vi "relay_block4.vi"(8 "error in":errorcluster, 11 "Modbus master in":refnum<class "Modbus Master.lvclass">) -> (0 "error out":errorcluster, 3 "Modbus master out":refnum<class "Modbus Master.lvclass">)   [LabVIEW 2020]
uses:
  <vilib>/NI/Modbus Library/API/Master/Modbus Master.lvclass
  C:/Program Files/National Instruments/LabVIEW 2020/vi.lib/NI/Modbus Library/API/Modbus API.lvclass
  <vilib>/NI/Modbus Library/API/Modbus API.lvclass/Modbus API.ctl
  <vilib>/NI/Modbus Library/Transmission Data Unit/Transmission Data Unit.lvclass/Transmission Data Unit.ctl
  <vilib>/NI/Modbus Library/Transmission Data Unit/Write Unit ID.vi
  <vilib>/NI/Modbus Library/API/Read Transmission Data Unit.vi
  <vilib>/NI/Modbus Library/API/Write Transmission Data Unit.vi
  status/emergency stop.vi
panel:
  out "current time 2":timestamp
  out "current time":timestamp
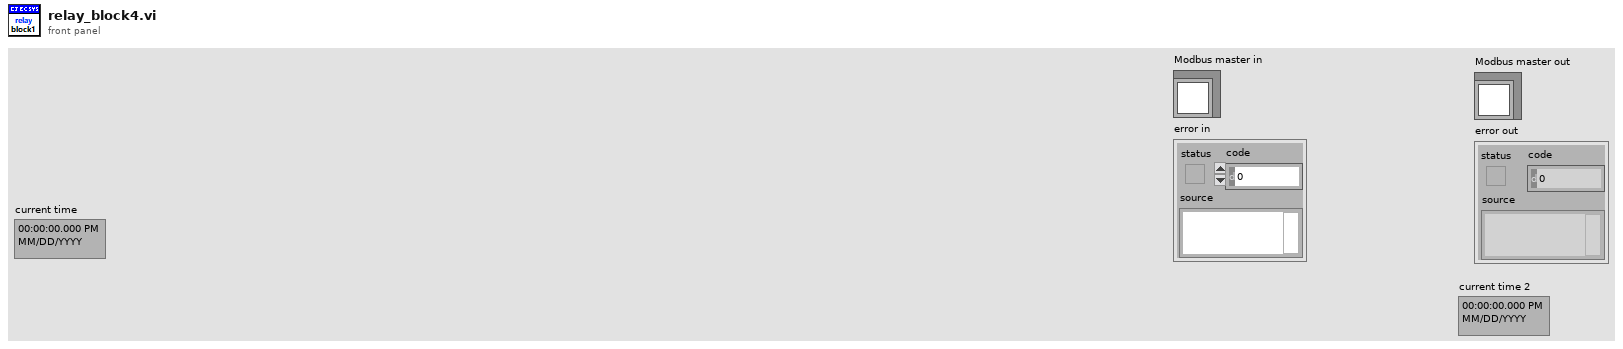
[diagram p1: front panel]
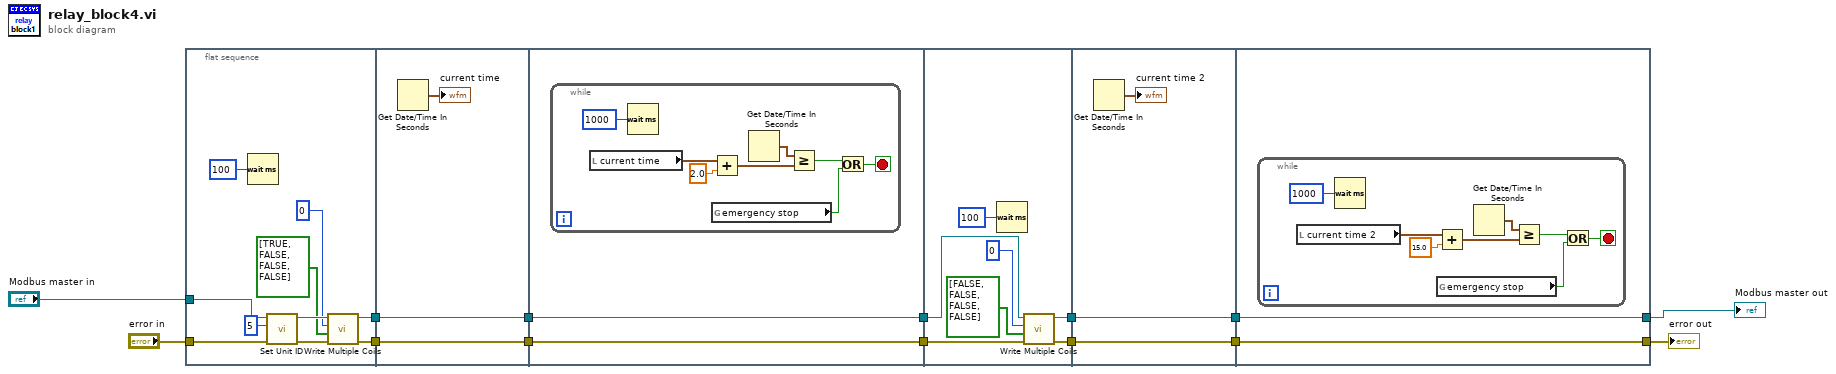
[diagram p0: block diagram]
diagram:
  n1 = flat-sequence {
    tunnel: "Modbus master in" -> [w19]
    tunnel: "error in" -> [w18]
    tunnel: [w17] -> w12
    tunnel: [w16] -> w7
    tunnel: w12 -> [w26]
    tunnel: [w26] -> w11
    tunnel: [w25] -> w8
    tunnel: w7 -> [w25]
    tunnel: w11 -> [w29]
    tunnel: [w29] -> w10
    tunnel: [w28] -> w9
    tunnel: w8 -> [w28]
    tunnel: w10 -> [w41]
    tunnel: w9 -> [w40]
    tunnel: [w39] -> w5
    tunnel: [w38] -> w2
    tunnel: [w46] -> w6
    tunnel: w5 -> [w46]
    tunnel: [w45] -> w3
    tunnel: w2 -> [w45]
    tunnel: w6 -> [w49]
    tunnel: [w49] -> w4
    tunnel: w3 -> [w48]
    tunnel: [w48] -> w1
    frame #0 {
      n2 = Wait (ms)(milliseconds to wait=u32 100 ("millisecond timer value")) -> ()  [unwired: 1 out]
      n3 = call <vilib>:"Set Unit ID.vi"("error in"=w18, "unit ID"=u8 5, "Modbus master in"=w19) -> ("error out"=w23:errorcluster, "Modbus master out"=w22:refnum<class "Modbus Master.lvclass">)  [unwired: 7 in]
      n4 = call-dynamic "Write Multiple Coils.vi"("error in"=w23, "coils to write"=bool[] [TRUE, FALSE, FALSE, FALSE] ("coils 2"), "starting address"=u16 0, "Modbus master in"=w22) -> ("error out"=w16:errorcluster, "Modbus master out"=w17:refnum<class "Modbus Master.lvclass">)  [unwired: 6 in]
    }
    frame #1 {
      n5 = Get Date/Time In Seconds() -> (seconds since 1Jan1904=→"current time":timestamp)
    }
    frame #2 {
      n6 = while {
        stop <- w30 stop-if-true
        n7 = local read "current time"() -> (w36:timestamp)
        n8 = Wait (ms)(milliseconds to wait=u32 1000 ("millisecond timer value")) -> ()  [unwired: 1 out]
        n9 = Add(x=w36, y=2.0) -> (x+y=w34:timestamp)
        n10 = global read "emergency stop.vi" "emergency stop"() -> (w31:bool)
        n11 = Get Date/Time In Seconds() -> (seconds since 1Jan1904=w33:timestamp)
        n12 = Greater Or Equal?(x=w33, y=w34) -> (x >= y?=w32:bool)
        n13 = Or(x=w32, y=w31) -> (x .or. y?=w30:bool)
      }
    }
    frame #3 {
      n14 = Wait (ms)(milliseconds to wait=u32 100 ("millisecond timer value")) -> ()  [unwired: 1 out]
      n15 = call-dynamic "Write Multiple Coils.vi"("error in"=w40, "coils to write"=bool[] [FALSE, FALSE, FALSE, FALSE] ("coils 2"), "starting address"=u16 0, "Modbus master in"=w41) -> ("error out"=w38:errorcluster, "Modbus master out"=w39:refnum<class "Modbus Master.lvclass">)  [unwired: 6 in]
    }
    frame #4 {
      n16 = Get Date/Time In Seconds() -> (seconds since 1Jan1904=→"current time 2":timestamp)
    }
    frame #5 {
      n17 = while {
        stop <- w50 stop-if-true
        n18 = local read "current time 2"() -> (w56:timestamp)
        n19 = Wait (ms)(milliseconds to wait=u32 1000 ("millisecond timer value")) -> ()  [unwired: 1 out]
        n20 = Add(x=w56, y=15.0) -> (x+y=w54:timestamp)
        n21 = global read "emergency stop.vi" "emergency stop"() -> (w51:bool)
        n22 = Get Date/Time In Seconds() -> (seconds since 1Jan1904=w53:timestamp)
        n23 = Greater Or Equal?(x=w53, y=w54) -> (x >= y?=w52:bool)
        n24 = Or(x=w52, y=w51) -> (x .or. y?=w50:bool)
      }
    }
  }
  "Modbus master out" <- w4
  "error out" <- w1
